vi "FRCts20_Backend_Comment_POST.vi"(6 "Message Attributes":T4, 8 "error in (no error)":errorcluster, 10 "Data":string, 11 "Engine_Refnums":T1) -> (0 "error out":errorcluster)   [LabVIEW 2014, in "FRCts20_Backend_Engine.lvlib"]
doc: "Adds a comment, called by the comment API. Expects a request index, author, and the note text. Returns the new comment's index"
uses:
  FRCts20_Backend_Engine.lvlib
  Dependencies/Keyed Array/KeyedArray.ctl
  FRCts20_Backend_EngineRefnums.ctl
  INI_Accessor/FRCts20_Backend_INI Controller.lvclass
  Dependencies/AMC/_SubVIs/TypeDefs/Message Queue.ctl
  Dependencies/AMC/_SubVIs/TypeDefs/Message.ctl
  <vilib>/addons/database/Connection.llb/Conn ObjectReference.ctl
  FRCts20_Backend_FGVOperation.ctl
  FRCts20_Backend_API/FRCts20_Backend_API_Note.ctl
  FRCts20_Backend_API/FRCts20_Backend_API.lvlib
  Dependencies/Keyed Array/Tools_KeyedArray.lvlib
  Dependencies/AMC/AMC.lvlib
  <vilib>/addons/database/NI_Database_API.lvlib
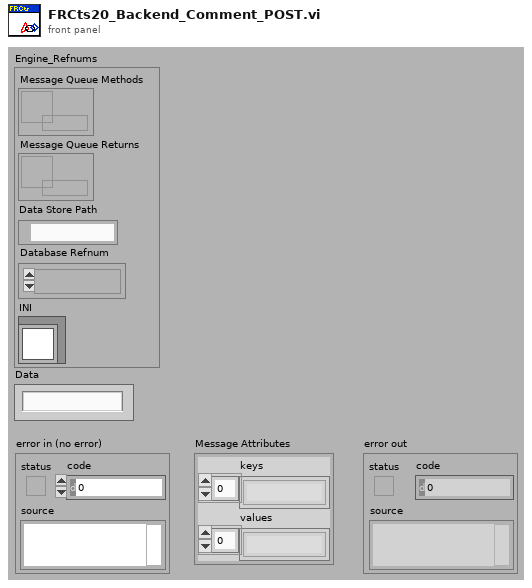
[diagram p1: front panel]
types:
  T1 = typedef "FRCts20_Backend_Engine.lvlib/FRCts20_Backend_EngineRefnums.ctl" = cluster{"Message Queue Methods":T2, "Message Queue Returns":T2, "Data Store Path":path, "Database Refnum":T3, "INI":refnum<class "FRCts20_Backend_INI Controller.lvclass">}
  T2 = typedef "AMC.lvlib/Message Queue.ctl" = refnum<queue>
  T3 = typedef "NI_Database_API.lvlib/Conn ObjectReference.ctl" = refnum<k1>
  T4 = typedef "Tools_KeyedArray.lvlib/KeyedArray.ctl" = cluster{"keys":string[], "values":string[]}
  T5 = typedef "FRCts20_Backend_API.lvlib/FRCts20_Backend_API_Note.ctl" = cluster{"Note Index":u32, "Request Index":u32, "Author":string, "Time Entered":timestamp, "Text":string, "Solution":bool, "APIReturn":string}
  T6 = typedef "FRCts20_Backend_Engine.lvlib/FRCts20_Backend_FGVOperation.ctl" = enum16{"Initialize", "EnqueueMessage", "EnqueueDataReturn", "FlushMessage", "FlushDataReturn"}
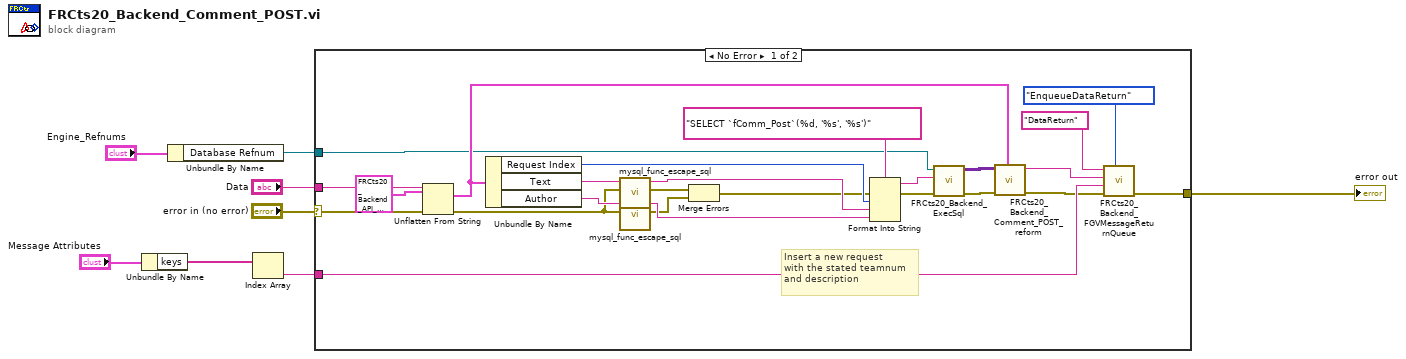
[diagram p0: block diagram]
diagram:
  n1 = Unbundle By Name("Message Attributes") -> ("keys"=w2:string[])
  n2 = Unbundle By Name("Engine_Refnums") -> ("Database Refnum"=w5:T3)
  n3 = Index Array(array=w2) -> (element=w1:string)  [unwired: 1 in]
  n4 = case shown="No Error" "error in (no error)" {
    selector: "error in (no error)" -> [w30 w34]
    tunnel: [w33 w34] -> w7
    tunnel: w5 -> [w13 _]
    tunnel: "Data" -> [w31 _]
    tunnel: w1 -> [w32 _]
    frame No Error {
      # "Insert a new request\nwith the stated teamnum\nand description"
      n5 = Unflatten From String(type=T5 {"Note Index"=0, "Request Index"=0, "Author"="", "Time Entered"=timestamp(0 s since 1904-01-01), "Text"="", "Solution"=FALSE, "APIReturn"=""} ("Note"), binary string=w31, error in (no error)=w30) -> (value=w18:T5, error out=w17:errorcluster)  [unwired: 2 in, 1 out]
      n6 = Unbundle By Name(w18) -> ("Request Index"=w23:u32, "Text"=w22:string, "Author"=w21:string)
      n7 = call "mysql_func_escape_sql.vi"("error in (no error)"=w17, "sqlin"=w22) -> ("error out"=w16:errorcluster, "escaped"=w20:string)  [unwired: 8 in]
      n8 = call "mysql_func_escape_sql.vi"("error in (no error)"=w17, "sqlin"=w21) -> ("error out"=w15:errorcluster, "escaped"=w19:string)  [unwired: 8 in]
      n9 = Merge Errors(w16, w15) -> (w14:errorcluster)
      n10 = Format Into String(format string="SELECT `fComm_Post`(%d, '%s', '%s')", error in=w14, w23, w20, w19) -> (resulting string=w12:string, error out=w11:errorcluster)  [unwired: 1 in]
      n11 = call "FRCts20_Backend_ExecSql.vi"("error in (no error)"=w11, "format string"=w12, "Refnum in"=w13) -> ("error out"=w10:errorcluster, "recordset data"=w9:variant[][])  [unwired: 6 in, 1 out]
      n12 = call "FRCts20_Backend_Comment_POST_reform.vi"("Note"=w18, "error in (no error)"=w10, "recordset data"=w9) -> ("error out"=w25:errorcluster, "data string"=w26:string)  [unwired: 7 in]
      n13 = call "FRCts20_Backend_FGVMessageReturnQueue.vi"("Operation"=FRCts20_Backend_FGVOperation."EnqueueDataReturn", "error in (no error)"=w25, "Key"=w32, "Message Value"=w26, "Message Name"="DataReturn") -> ("error out"=w33:errorcluster)  [unwired: 5 in, 1 out]
    }
    frame Error {
    }
  }
  "error out" <- w7
